vi "KE622x -- 2182 -A Get Digital Filter Type.vi"(0 "622x Resource In":refnum<visa-resource-name>, 1 "Check For SCPI Errors? (T)":bool=TRUE, 11 "error in (no error)":errorcluster) -> (4 "622x Resource Out (dupl)":refnum<visa-resource-name>, 8 "Filter Type":enum16{"Movin", "Repeat"}(ring), 15 "error out":errorcluster)   [LabVIEW 2013, in "Keithly user program.lvlib"]
uses:
  Keithly user program.lvlib
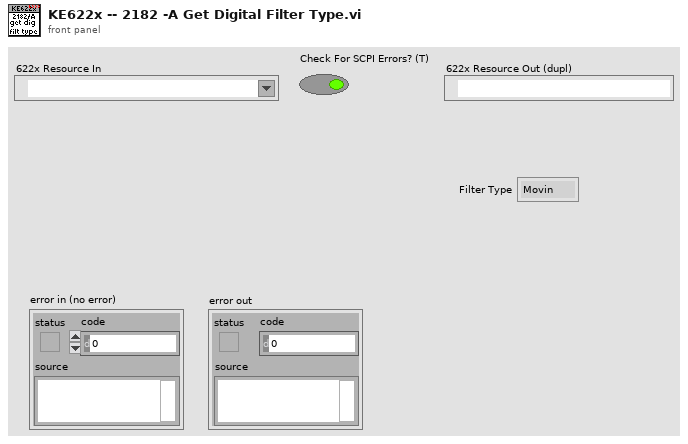
[diagram p1: front panel]
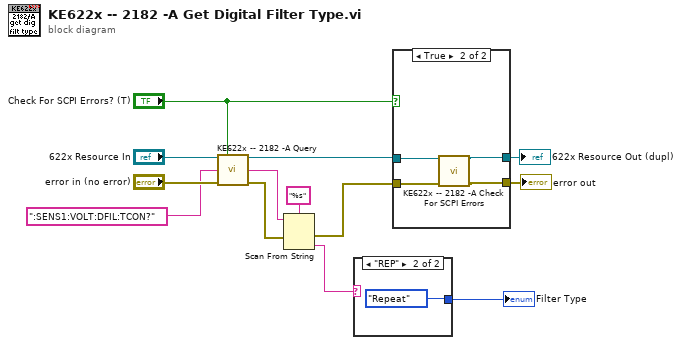
[diagram p0: block diagram]
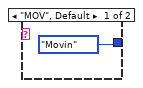
[diagram p2: hidden frame]
diagram:
  n1 = call "KE622x -- 2182 -A Query.vi"("622x Resource In"="622x Resource In", "Check For SCPI Errors? (T)"="Check For SCPI Errors? (T)", "2182-A Write String"=":SENS1:VOLT:DFIL:TCON?", "error in (no error)"="error in (no error)") -> ("622x Resource Out (dupl)"=w6:refnum<visa-resource-name>, "2182-A Reponse String"=w3:string, "error out"=w2:errorcluster)  [unwired: 9 in]
  n2 = Scan From String(format string="%s", input string=w3, error in=w2) -> (error out=w12:errorcluster, output 1=w9:string)  [unwired: 2 in, 2 out]
  n3 = case shown="\"REP\"" w9 {
    tunnel: [enum16{"Movin", "Repeat"}."Movin" ("Filter Type") enum16{"Movin", "Repeat"}."Repeat" ("Filter Type")] -> w1
    frame "MOV", Default {
    }
    frame "REP" {
    }
  }
  "Filter Type" <- w1
  n4 = case shown="True" "Check For SCPI Errors? (T)" {
    tunnel: w6 -> [w17 w21]
    tunnel: w12 -> [w16 w19]
    tunnel: [w17 w20] -> w11
    tunnel: [w16 w18] -> w10
    frame False {
    }
    frame True {
      n5 = call "KE622x -- 2182 -A Check For SCPI Errors.vi"("VISA Resource In"=w21, "error in (no error)"=w19) -> ("VISA Resource Out (dupl)"=w20:refnum<visa-resource-name>, "error out"=w18:errorcluster)  [unwired: 10 in, 2 out]
    }
  }
  "622x Resource Out (dupl)" <- w11
  "error out" <- w10
